vi "contagem_gauge.vi"() -> ()   [LabVIEW 2018]
uses:
  <vilib>/Instr/_visa.llb/VISA Configure Serial Port (Instr).vi
panel:
  in  "stop":bool
  out "Gauge":dbl(knob) scale=0.0..100.0
  in  "VISA resource name":refnum<visa-resource-name>
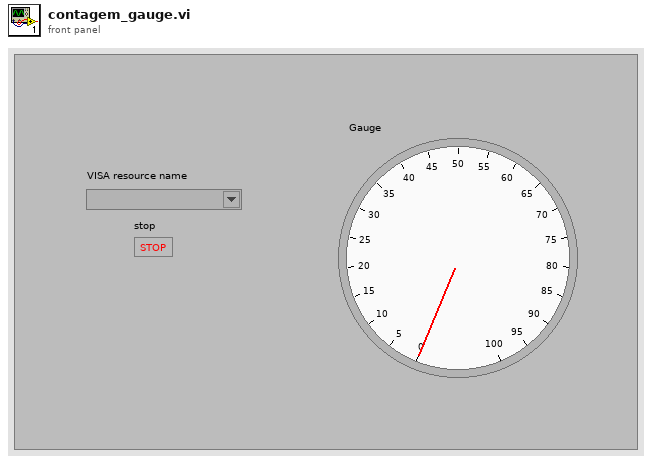
[diagram p1: front panel]
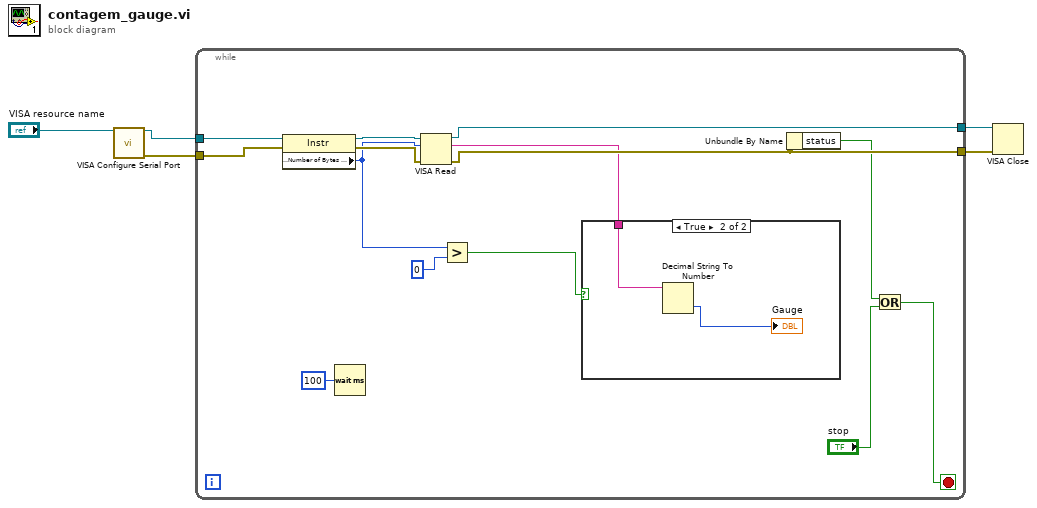
[diagram p0: block diagram]
diagram:
  n1 = call-poly "VISA Configure Serial Port"("VISA resource name"="VISA resource name") -> ("VISA resource name out"=w4:refnum<visa-resource-name>, "error out"=w3:errorcluster)  [unwired: 13 in]
  n2 = while {
    tunnel: w4 -> [w18]
    tunnel: w3 -> [w17]
    tunnel: [w10] -> w2
    tunnel: [w11] -> w1
    stop <- w8 stop-if-true
    n3 = property class="Instr"(reference=w18, error in=w17) -> (reference out=w15:refnum<visa-resource-name>, error out=w16:errorcluster, "Serial Settings:Number of Bytes at Serial Port"=w14:u32)
    n4 = Wait (ms)(milliseconds to wait=u32 100) -> ()  [unwired: 1 out]
    n5 = VISA Read(VISA resource name=w15, byte count=w14, error in (no error)=w16) -> (VISA resource name out=w11:refnum<visa-resource-name>, read buffer=w6:string, error out=w10:errorcluster)  [unwired: 1 out]
    n6 = Greater?(x=w14, y=u32 0) -> (0:w12:bool)
    n7 = case shown="True" w12 {
      tunnel: w6 -> [_ w21]
      frame False {
      }
      frame True {
        n8 = Decimal String To Number(string=w21) -> (number=→"Gauge":i32)  [unwired: 2 in, 1 out]
      }
    }
    n9 = Unbundle By Name(w10) -> ("status"=w9:bool)
    n10 = Or(x=w9, y="stop") -> (x .or. y?=w8:bool)
  }
  n11 = VISA Close(VISA resource name=w1, error in (no error)=w2) -> ()  [unwired: 1 out]
